vi "BK Precision 9115.vi"() -> ()   [LabVIEW 2020]
uses:
  LabVIEW 2020 Toolkits/toolkits_lv2020_32bit/Synchronization.llb/SynchRefs_SetGet.ctl
  LabVIEW 2020 Toolkits/VI Server Toolkit/VI Server Libraries/VI Server_Set Controls.llb/Set STR Control.vi
  LabVIEW 2020 Toolkits/VI Server Toolkit/VI Server Libraries/VI Server_SetControl.llb/VI Server_BOOL_Set.vi
  LabVIEW 2020 Toolkits/VI Server Toolkit/VI Server Toolkit LV2013.lvlib
panel:
  out "System.Message":string caption="System Message"
  in  "Help":bool
  in  "FP.Hide":bool caption="FrontPanel.Hide"
  in  "EXIT":bool
  in  "error in":errorcluster
  in  "Tab.Main":T1(tab)
  out "Indicator.List.Running":bool
  in  "Indicator.OVP.Level.Measured":dbl caption="Vovp =" format="%0.3f V"
  in  "Indicator.Power.Measured":dbl format="%0.1fW"
  in  "Indicator.Current.Measured":dbl format="%0.3fA"
  in  "Indicator.Voltage.Measured":dbl format="%0.3fV"
  out "Indicator.Prot":bool
  out "Indicator.Trig":bool
  out "Indicator.Error":bool
  out "Indicator.Addr":bool
  out "Indicator.Rmt":bool
  out "Indicator.CC":bool
  out "Indicator.Output.Enabled":bool
  out "Indicator.CV":bool
  in  "OVP.Delay":dbl=0.001 caption="OVP.Delay.DUP" min=0.001 max=0.6 format="%0.3f sec"
  in  "OVP.Level":dbl caption="OVP.Level.DUP" min=0.0 max=80.0 format="%0.3f V"
  in  "Output.Amps":dbl caption="Output.Amps.DUP" min=0.0 max=80.0 format="%0.3f A"
  in  "Output.Volts":dbl caption="Output.Volts.DUP" min=0.0 max=80.0 format="%0.3f V"
  in  "*RST":bool
  in  "LOCAL":bool
  in  "OVP.Clear":bool
  in  "OVP.Enable":bool
  in  "OVP.Delay.DUP":dbl(knob)=0.001 caption="Protection Delay (sec)" min=0.001 max=0.6 scale=0.0..0.6
  in  "OVP.Level.DUP":dbl(knob) caption="Volts" min=0.0 max=80.0 scale=0.0..80.0
  in  "Output.Enable":bool
  in  "Output.Amps.DUP":dbl(knob) caption="Current Limit (Amp)" scale=0.0..60.0
  in  "Output.Volts.DUP":dbl(knob) caption="Volts" min=0.0 max=80.0 scale=0.0..80.0
  in  "Sequence.ActiveSteps":bool[](array[boolean]) caption="Active Steps"
  in  "List.LinkedSequences":bool[](array[boolean]) caption="Linked Sequences"
  in  "List.File.RUN":bool
  in  "Sequence.Load":bool
  in  "Sequence.Save":bool caption="List.File.Save"
  in  "Sequence.RepeatCount":u16[](array[numeric]) caption="Sequence Repeat Count" min=1
  in  "List.RepeatCount":u16=1 caption="List Repeat Count" min=1
  in  "List.PowerLimit":dbl=1.0 caption="List Power Limit" min=1.0 max=1200.0 format="%0.2f W"
  in  "List.File.Load":bool
  in  "List.File.Save":bool
  in  "List.File":u16=1 caption="List File" min=1 max=10
  in  "Sequence.Number":u16=1 caption="Sequence Number" min=1 max=10
  in  "Step.Parameters":T2(array[cluster]) caption="Step Parameters" {"Step.Slope" min=0.01 max=65.535 format="%0.2f sec"; "Step.Width" min=0.001 max=65.535 format="%0.3f sec"; "Step.Current" format="%0.3f A"; "Step.Voltage" format="%0.3f V"}
  out "Sequence.Graph":cluster{i32[], dbl[]}[](graph)
  out "VISA.Messages.Errors":string[](array[string]) caption="VISA Messages Errors"
  in  "Measurements.AutoUpdate.Disable":bool
  in  "Measurements.UpdateRate":u32=100 caption="Measurements Update Rate" min=100 max=100000 format="%.0f msec"
  in  "VISA.Command2.Write":bool
  in  "VISA.Command2":string caption="Command"
  in  "VISA.Command.Write":bool
  in  "VISA.Command":string caption="Command"
  out "VISA.InstrumentResponce":string caption="Instrument Responce"
  in  "VISA.ResourceName":refnum<visa-resource-name>="BK_PRECISION_9115" caption="VISA Rresource Name"
  in  "UDP.Test.String2.Send":bool
  in  "UDP.Test.String2":string caption="UDP: Test String 2"
  in  "UDP.Port.Receiver":u16=58433 caption="UDP: Port.Receiver"
  in  "UDP.Port.Read":u16=58432 caption="UDP: Port.Read"
  in  "UDP.LocalPort.Write":u16=58434 caption="UDP: Local Port.Write"
  in  "UDP.IP.Address":string="234.5.6.7" caption="UDP: IP Address"
  in  "UDP.Test.String1.Send":bool
  in  "UDP.Test.String1":string caption="UDP: Test String 1"
  in  "UDP.Responce.String.Monitor":bool
  out "UDP.Responce.String":string caption="UDP: Responce String"
  in  "VI.WindowsTitle":string caption="Windows Title"
  out "error out":errorcluster={"status"=TRUE, "code"=1055, "source"="Property Node in VI Server Toolkit LV2013.lvlib:VI server_Set Control Value from String Format.vi:5200001->DMM6500_UDP_ExecEng_Instruction_APPLY.vi->DMM6500_UDP_MAIN.vi->Keithley2100.vi"}
  # "OVERVOLTAGE"
  # "OUTPUT"
  # "Seqience Setup"
  # "Step #         Voltage              Current                  Width                     Slope"
  # "1\n\n\n\n2\n\n\n\n3\n\n\n4\n\n\n\n5\n\n\n\n6\n\n\n\n7\n\n\n8\n\n\n\n9\n\n\n\n10"
  # "1       2       3       4       5      6       7      8       9      10"
  # "1       2       3       4       5      6       7      8       9      10"
  # "1"
  # "2"
  # "3"
  # "4"
  # "5"
  # "6"
  # "7"
  # "8"
  # "9"
  # "10"
  # "Multicast IP addresses must be in the 224.0.0.0 to 239.255.255.255 range."
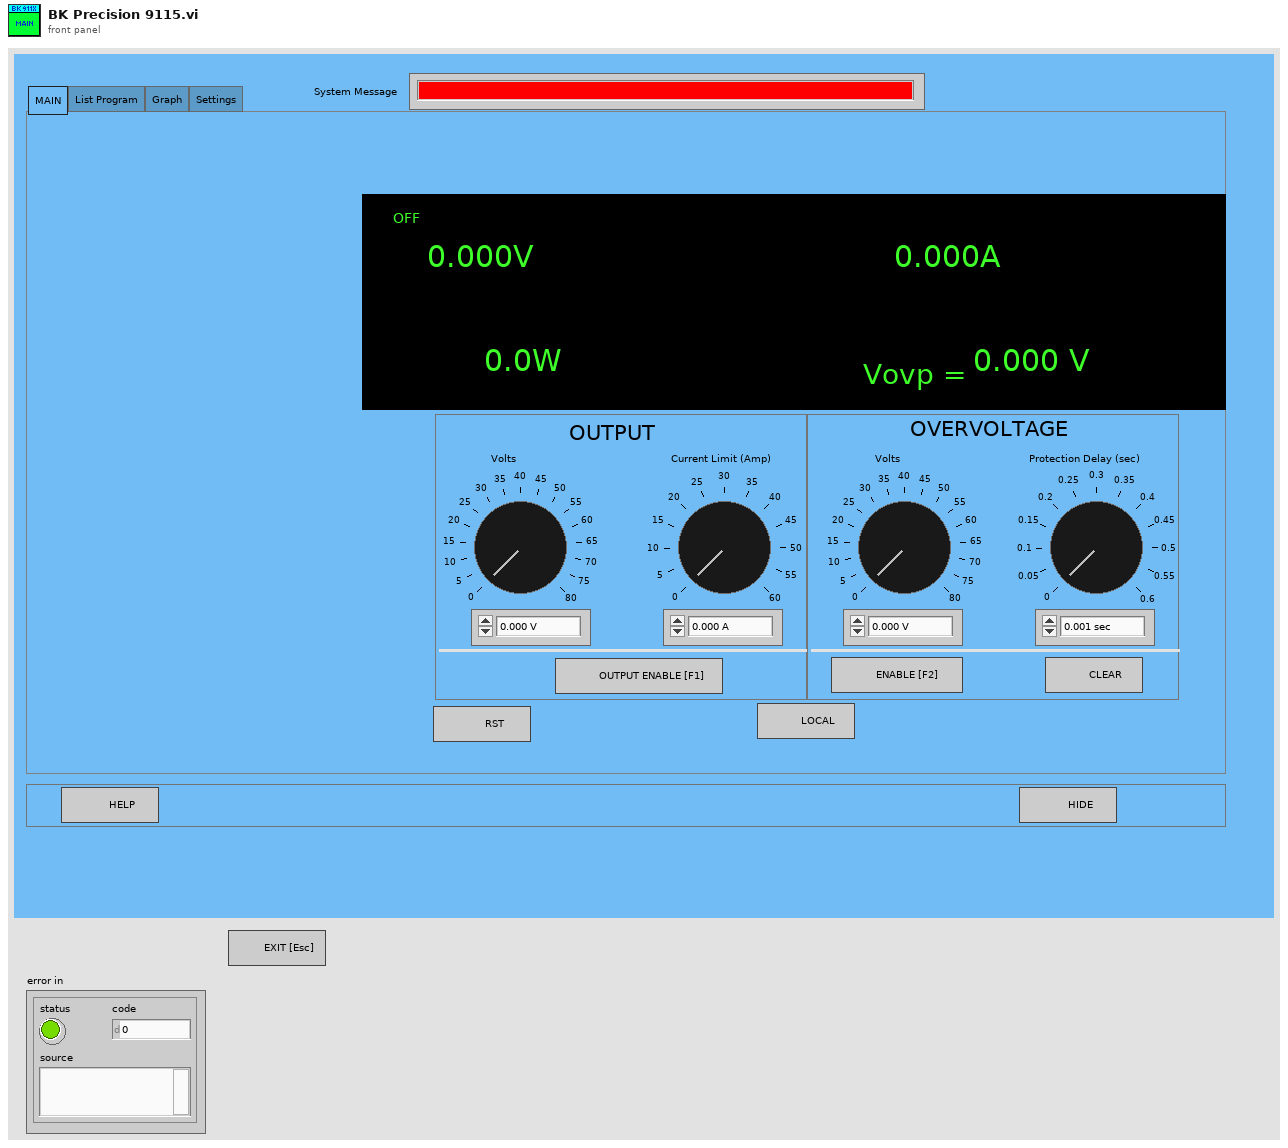
[diagram p1: front panel]
types:
  T1 = enum32{"MAIN", "List Program", "Graph", "Settings"}
  T2 = cluster{"Step.Voltage":dbl, "Step.Current":dbl, "Step.Width":dbl, "Step.Slope":dbl}[]
  T3 = typedef "VI Server_RefsCluster.ctl" = cluster{"Labels":string[], "Refs":refnum<vi>[], "VI Ref":refnum<vi>}
  T4 = typedef "SynchRefs_SetGet.ctl" = enum16{"Set", "Get"}
  T5 = typedef "Semaphore RefNum" = refnum<k1>
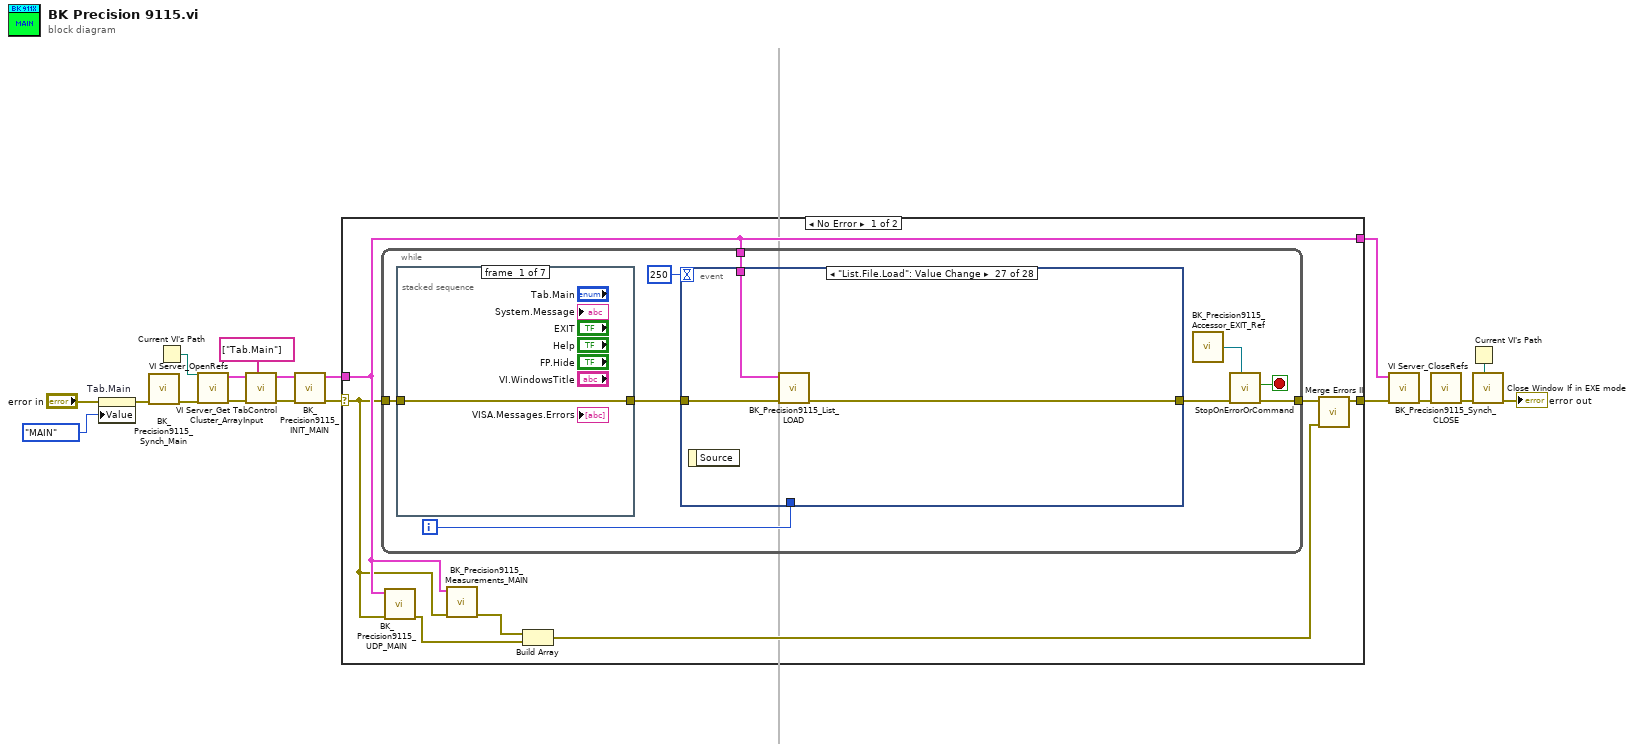
[diagram p0: block diagram]
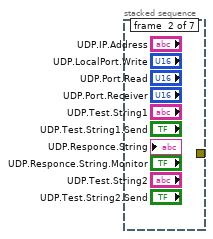
[diagram p2: hidden frame]
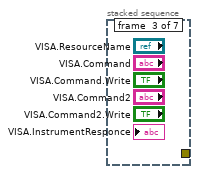
[diagram p3: hidden frame]
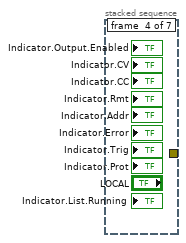
[diagram p4: hidden frame]
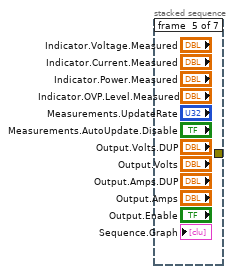
[diagram p5: hidden frame]
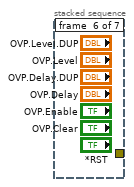
[diagram p6: hidden frame]
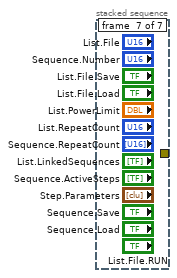
[diagram p7: hidden frame]
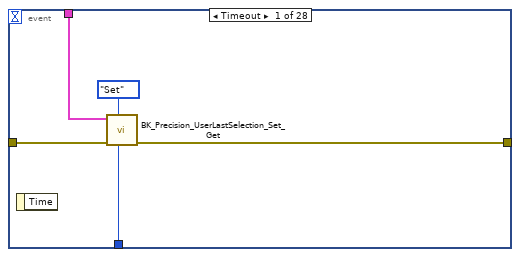
[diagram p8: hidden frame]
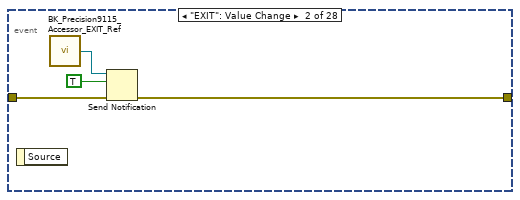
[diagram p9: hidden frame]
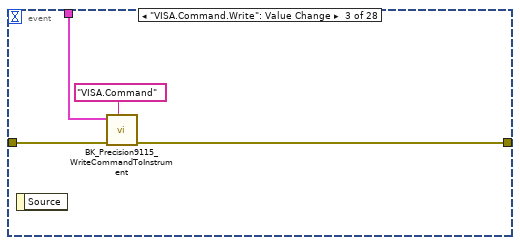
[diagram p10: hidden frame]
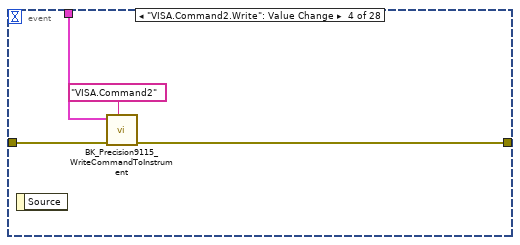
[diagram p11: hidden frame]
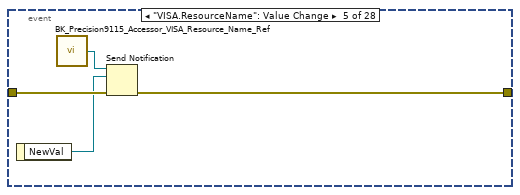
[diagram p12: hidden frame]
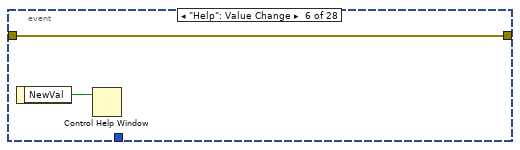
[diagram p13: hidden frame]
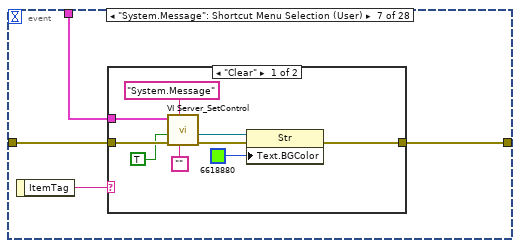
[diagram p14: hidden frame]
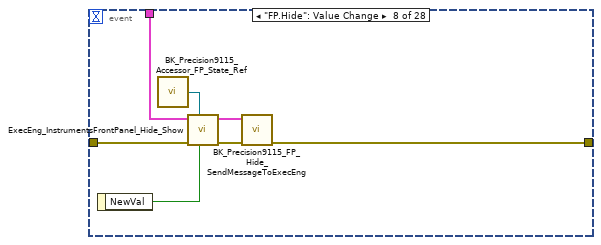
[diagram p16: hidden frame]
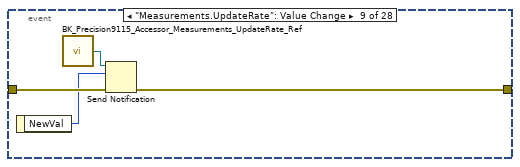
[diagram p17: hidden frame]
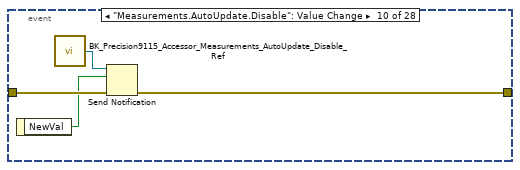
[diagram p18: hidden frame]
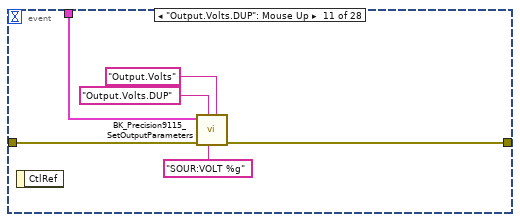
[diagram p19: hidden frame]
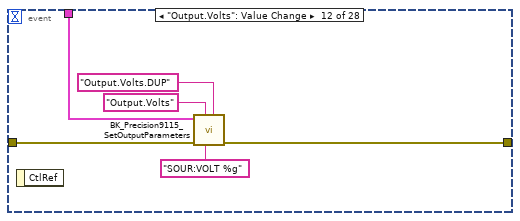
[diagram p20: hidden frame]
diagram:
  n1 = property on="Tab.Main" class="TabCtl (strict)"(error in="error in", "Value"=T1."MAIN" ("Tab.Main")) -> (error out=w2:errorcluster)  [unwired: 1 in, 1 out]
  n2 = call "BK_Precision9115_Synch_Main.vi"("error in"=w2) -> ("error out"=w15:errorcluster)  [unwired: 10 in]
  n3 = Current VI's Path() -> (path=w17:path)
  n4 = call "VI Server_OpenRefs.vi"("error in"=w15, "VI Path"=w17) -> ("error out"=w14:errorcluster, "VI Server.RefsCluster"=w16:T3)  [unwired: 8 in]
  n5 = call "VI Server_Get TabControl Cluster_ArrayInput.vi"("TabControl Labels[]"=string[] ["Tab.Main"], "error in"=w14, "VI Server Cluster"=w16) -> ("error out"=w9:errorcluster, "VI Server Cluster.OUT"=w8:T3)  [unwired: 7 in]
  n6 = call "BK_Precision9115_INIT_MAIN.vi"("error in (no error)"=w9, "VI Server Cluster"=w8) -> ("error out"=w7:errorcluster, "VI Server Cluster DUP"=w5:T3)  [unwired: 8 in]
  n7 = case shown="No Error" w7 {
    selector: w7 -> [w22 w189]
    tunnel: [w24 w189] -> w6
    tunnel: w5 -> [w23 w188]
    tunnel: [w23 w188] -> w4
    frame No Error {
      n8 = while {
        tunnel: w22 -> [w34]
        tunnel: w23 -> [w31]
        tunnel: [w27] -> w25
        i -> [w30]
        stop <- w26 stop-if-true
        n9 = stacked-sequence {
          tunnel: w34 -> [w35 _ _ _ _ _ _]
          tunnel: [w35 _ _ _ _ _ _] -> w32
          frame #0 {
          }
          frame #1 {
          }
          frame #2 {
          }
          frame #3 {
          }
          frame #4 {
          }
          frame #5 {
          }
          frame #6 {
          }
        }
        n10 = event shown="[26] \"List.File.Load\": Value Change" {
          selector: _ -> [_ _ _ _ _ _ _ _ _ _ _ _ _ _ _ _ _ _ _ _ _ _ _ _ _ _ _ _]
          dyn-events: _ -> [_ _ _ _ _ _ _ _ _ _ _ _ _ _ _ _ _ _ _ _ _ _ _ _ _ _ _ _]
          timeout: 250 -> [_ _ _ _ _ _ _ _ _ _ _ _ _ _ _ _ _ _ _ _ _ _ _ _ _ _ _ _]
          tunnel: w32 -> [w40 w44 w48 w52 w56 w57 w61 w79 w83 w87 w92 w98 w104 w110 w114 w120 w126 w132 w138 w143 w146 w159 w171 w174 w177 w180 w183 w187]
          tunnel: w31 -> [w39 _ w47 w51 _ _ w59 w77 _ _ w91 w97 w103 w109 w113 w119 w125 w131 w137 w141 w144 w161 w169 w173 w175 w179 w181 w186]
          tunnel: [w36 w42 w46 w50 w53 w57 w60 w74 w80 w85 w93 w99 w105 w111 w115 w121 w127 w133 w139 w142 w147 w163 w170 w172 w176 w178 w182 w185] -> w28
          tunnel: w30 -> [w38 _ _ _ _ _ _ _ _ _ _ _ _ _ _ _ _ _ _ _ _ _ _ _ _ _ _ _]
          event Timeout {
            n11 = event-data() -> ()  [unwired: 1 in, 1 out]
            n12 = call "BK_Precision_UserLastSelection_Set_Get.vi"("LoopCounter"=w38, "SynchRefs.Set/Get"=SynchRefs_SetGet."Set", "error in"=w40, "VI Server.RefsCluster"=w39) -> ("error out"=w36:errorcluster)  [unwired: 6 in, 1 out]
          }
          event "EXIT": Value Change {
            n13 = event-data() -> ()  [unwired: 1 in, 1 out]
            n14 = call "BK_Precision9115_Accessor_EXIT_Ref.vi"() -> ("EXIT"=w43:refnum<notifier>)  [unwired: 6 in]
            n15 = Send Notification(notification=TRUE, notifier=w43, error in (no error)=w44) -> (error out=w42:errorcluster)  [unwired: 1 out]
          }
          event "VISA.Command.Write": Value Change {
            n16 = event-data() -> ()  [unwired: 1 in, 1 out]
            n17 = call "BK_Precision9115_WriteCommandToInstrument.vi"("Control.Label"="VISA.Command", "error in (no error)"=w48, "VI Server Cluster"=w47) -> ("error out"=w46:errorcluster)  [unwired: 8 in]
          }
          event "VISA.Command2.Write": Value Change {
            n18 = event-data() -> ()  [unwired: 1 in, 1 out]
            n19 = call "BK_Precision9115_WriteCommandToInstrument.vi"("Control.Label"="VISA.Command2", "error in (no error)"=w52, "VI Server Cluster"=w51) -> ("error out"=w50:errorcluster)  [unwired: 8 in]
          }
          event "VISA.ResourceName": Value Change {
            n20 = event-data() -> ("NewVal"=w54:refnum<visa-resource-name>)  [unwired: 1 in]
            n21 = call "BK_Precision9115_Accessor_VISA_Resource_Name_Ref.vi"() -> ("VISA resource name"=w55:refnum<notifier>)  [unwired: 6 in]
            n22 = Send Notification(notification=w54, notifier=w55, error in (no error)=w56) -> (error out=w53:errorcluster)  [unwired: 1 out]
          }
          event "Help": Value Change {
            n23 = event-data() -> ("NewVal"=w58:bool)  [unwired: 1 in]
            n24 = Control Help Window(1:w58) -> ()  [unwired: 1 in]
          }
          event "System.Message": Shortcut Menu Selection (User) {
            n25 = event-data() -> ("ItemTag"=w62:string)  [unwired: 1 in]
            n26 = case shown="\"Clear\"" w62 {
              tunnel: w61 -> [w67 w72]
              tunnel: [w68 w72] -> w60
              tunnel: w59 -> [w65 _]
              frame "Clear" {
                n27 = call-poly "VI Server_SetControl.vi"("New Value"="", "Label"="System.Message", "error in"=w67, "Single Instance (T)"=TRUE ("SingleInstance"), "VI Server Cluster"=w65) -> ("error out"=w70:errorcluster, "Control Ref"=w71:refnum<vi>)  [unwired: 4 in, 1 out]
                n28 = property class="Str"(reference=w71, error in=w70, "Text.BGColor"=u32 6618880) -> (error out=w68:errorcluster)  [unwired: 1 out]
              }
              frame "", Default {
              }
            }
          }
          event "FP.Hide": Value Change {
            n29 = event-data() -> ("NewVal"=w78:bool)  [unwired: 1 in]
            n30 = call "BK_Precision9115_Accessor_FP_State_Ref.vi"() -> ("FP.State"=w76:refnum<notifier>)  [unwired: 6 in]
            n31 = call "ExecEng_InstrumentsFrontPanel_Hide_Show.vi"("FP.Hide/Show"=w78, "FP.State"=w76, "error in (no error)"=w79, "VI Server Cluster"=w77) -> ("error out"=w75:errorcluster, "VI Server Cluster DUP"=w73:T3)  [unwired: 6 in]
            n32 = call "BK_Precision9115_FP_Hide_SendMessageToExecEng.vi"("error in (no error)"=w75, "VI Server Cluster"=w73) -> ("error out"=w74:errorcluster)  [unwired: 9 in]
          }
          event "Measurements.UpdateRate": Value Change {
            n33 = event-data() -> ("NewVal"=w81:u32)  [unwired: 1 in]
            n34 = call "BK_Precision9115_Accessor_Measurements_UpdateRate_Ref.vi"() -> ("Measurements.UpdateRate"=w82:refnum<notifier>)  [unwired: 6 in]
            n35 = Send Notification(notification=w81, notifier=w82, error in (no error)=w83) -> (error out=w80:errorcluster)  [unwired: 1 out]
          }
          event "Measurements.AutoUpdate.Disable": Value Change {
            n36 = event-data() -> ("NewVal"=w86:bool)  [unwired: 1 in]
            n37 = call "BK_Precision9115_Accessor_Measurements_AutoUpdate_Disable_Ref.vi"() -> ("Measurements.AutoUpdate.Disable"=w84:refnum<notifier>)  [unwired: 6 in]
            n38 = Send Notification(notification=w86, notifier=w84, error in (no error)=w87) -> (error out=w85:errorcluster)  [unwired: 1 out]
          }
          event "Output.Volts.DUP": Mouse Up {
            n39 = event-data() -> ()  [unwired: 1 in, 1 out]
            n40 = call "BK_Precision9115_SetOutputParameters.vi"("DuplicateControl.Label"="Output.Volts" ("Control.Label"), "Command.Template"="SOUR:VOLT %g" ("Set Voltage"), "Control.Label"="Output.Volts.DUP", "error in (no error)"=w92, "VI Server Cluster"=w91) -> ("error out"=w93:errorcluster)  [unwired: 5 in, 1 out]
          }
          event "Output.Volts": Value Change {
            n41 = event-data() -> ()  [unwired: 1 in, 1 out]
            n42 = call "BK_Precision9115_SetOutputParameters.vi"("DuplicateControl.Label"="Output.Volts.DUP" ("Control.Label"), "Command.Template"="SOUR:VOLT %g" ("Set Voltage"), "Control.Label"="Output.Volts", "error in (no error)"=w98, "VI Server Cluster"=w97) -> ("error out"=w99:errorcluster)  [unwired: 5 in, 1 out]
          }
          event "Output.Amps.DUP": Mouse Up {
            n43 = event-data() -> ()  [unwired: 1 in, 1 out]
            n44 = call "BK_Precision9115_SetOutputParameters.vi"("DuplicateControl.Label"="Output.Amps" ("Control.Label"), "Command.Template"="SOUR:CURR %g" ("Set Voltage"), "Control.Label"="Output.Amps.DUP", "error in (no error)"=w104, "VI Server Cluster"=w103) -> ("error out"=w105:errorcluster)  [unwired: 5 in, 1 out]
          }
          event "Output.Amps": Value Change {
            n45 = event-data() -> ()  [unwired: 1 in, 3 out]
            n46 = call "BK_Precision9115_SetOutputParameters.vi"("DuplicateControl.Label"="Output.Amps.DUP" ("Control.Label"), "Command.Template"="SOUR:CURR %g" ("Set Voltage"), "Control.Label"="Output.Amps", "error in (no error)"=w110, "VI Server Cluster"=w109) -> ("error out"=w111:errorcluster)  [unwired: 5 in, 1 out]
          }
          event "Output.Enable": Value Change {
            n47 = event-data() -> ("NewVal"=w112:bool)  [unwired: 1 in]
            n48 = call "BK_Precision9115_Output_ENABLE.vi"("Output.Enable"=w112, "error in (no error)"=w114, "VI Server Cluster"=w113) -> ("error out"=w115:errorcluster)  [unwired: 8 in]
          }
          event "OVP.Level.DUP": Mouse Up {
            n49 = event-data() -> ()  [unwired: 1 in, 1 out]
            n50 = call "BK_Precision9115_SetOutputParameters.vi"("DuplicateControl.Label"="OVP.Level" ("Control.Label"), "Command.Template"="SOUR:VOLT:PROT %g" ("Set Voltage"), "Control.Label"="OVP.Level.DUP", "error in (no error)"=w120, "VI Server Cluster"=w119) -> ("error out"=w121:errorcluster)  [unwired: 5 in, 1 out]
          }
          event "OVP.Level": Value Change {
            n51 = event-data() -> ()  [unwired: 1 in, 1 out]
            n52 = call "BK_Precision9115_SetOutputParameters.vi"("DuplicateControl.Label"="OVP.Level.DUP" ("Control.Label"), "Command.Template"="SOUR:VOLT:PROT %g" ("Set Voltage"), "Control.Label"="OVP.Level", "error in (no error)"=w126, "VI Server Cluster"=w125) -> ("error out"=w127:errorcluster)  [unwired: 5 in, 1 out]
          }
          event "OVP.Delay.DUP": Mouse Up {
            n53 = event-data() -> ()  [unwired: 1 in, 1 out]
            n54 = call "BK_Precision9115_SetOutputParameters.vi"("DuplicateControl.Label"="OVP.Delay" ("Control.Label"), "Command.Template"="SOUR:VOLT:PROT:DEL %g" ("Set Voltage"), "Control.Label"="OVP.Delay.DUP", "error in (no error)"=w132, "VI Server Cluster"=w131) -> ("error out"=w133:errorcluster)  [unwired: 5 in, 1 out]
          }
          event "OVP.Delay": Value Change {
            n55 = event-data() -> ()  [unwired: 1 in, 1 out]
            n56 = call "BK_Precision9115_SetOutputParameters.vi"("DuplicateControl.Label"="OVP.Delay.DUP" ("Control.Label"), "Command.Template"="SOUR:VOLT:PROT:DEL %g" ("Set Voltage"), "Control.Label"="OVP.Delay", "error in (no error)"=w138, "VI Server Cluster"=w137) -> ("error out"=w139:errorcluster)  [unwired: 5 in, 1 out]
          }
          event "OVP.Enable": Value Change {
            n57 = event-data() -> ("NewVal"=w140:bool)  [unwired: 1 in]
            n58 = call "BK_Precision9115_OverVoltageProtection_Enable.vi"("OVP.Enable"=w140, "error in (no error)"=w143, "VI Server Cluster"=w141) -> ("error out"=w142:errorcluster)  [unwired: 8 in]
          }
          event "LOCAL": Value Change {
            n59 = event-data() -> ("NewVal"=w145:bool)  [unwired: 1 in]
            n60 = call "BK_Precision9115_Control_Local.vi"("Local"=w145, "error in (no error)"=w146, "VI Server Cluster"=w144) -> ("error out"=w147:errorcluster)  [unwired: 8 in]
          }
          event "*RST": Value Change {
            w152 = "*RST;*CLS" ("Set Voltage")
            n61 = event-data() -> ()  [unwired: 1 in, 1 out]
            n62 = call-poly "VI Server_SetControl.vi"("Data"=FALSE, "Control.Label"="*RST" ("Set Voltage"), "error in"=w159, "SingleInstance"=TRUE, "VI Server.RefsCluster"=w161) -> ("error out"=w160:errorcluster, "VI Server.RefsCluster.DUP"=w154:T3)  [unwired: 4 in, 1 out]
            n63 = call "BK_Precision9115_Accessor_VISA_Resource_Name_Ref.vi"() -> ("VISA resource name"=w168:refnum<notifier>)  [unwired: 6 in]
            n64 = call "BK_Precision9115_Accessor_Command.Sem_Ref.vi"() -> ("Command.Sem"=w164:T5)  [unwired: 6 in]
            n65 = call "Semaphore_Acquire.vi"("error in"=w160, "SemaphoreRef"=w164) -> ("error out"=w166:errorcluster)  [unwired: 8 in, 1 out]
            n66 = Get Notifier Status(notifier=w168, error in (no error)=w166) -> (current notification=w167:refnum<visa-resource-name>, error out=w165:errorcluster)  [unwired: 3 out]
            n67 = call "VISA WriteMod.vi"("error in"=w165, "String"=w152, "VISA resource name"=w167) -> ("error out"=w155:errorcluster, "VISA resource name DUP"=w153:refnum<visa-resource-name>)  [unwired: 6 in, 1 out]
            n68 = Current VI's Path() -> (path=w151:path)
            n69 = call "BK_Precision9115_ErrorHandler.vi"("Calling VI.Path"=w151, "Command"=w152, "VISA Refnum"=w153, "error in (no error)"=w155, "VI Server.RefsCluster"=w154) -> ("error out"=w149:errorcluster)  [unwired: 4 in, 2 out]
            n70 = call "BK_Precision9115_Accessor_Command.Sem_Ref.vi"() -> ("Command.Sem"=w162:T5)  [unwired: 6 in]
            n71 = call "Error 1073807246_SerialInterface_VISA resourceIsValidButNotAccessable.vi"("ShowError"=TRUE, "error in"=w149) -> ("error out"=w148:errorcluster)  [unwired: 12 in, 1 out]
            n72 = call "Semaphore_Release.vi"("error in"=w148, "SemaphoreRef"=w162) -> ("error out"=w163:errorcluster)  [unwired: 8 in, 1 out]
          }
          event "OVP.Clear": Value Change {
            n73 = event-data() -> ()  [unwired: 1 in, 1 out]
            n74 = call "BK_Precision9115_OVP_CLEAR.vi"("error in (no error)"=w171, "VI Server Cluster"=w169) -> ("error out"=w170:errorcluster)  [unwired: 8 in, 1 out]
          }
          event "Sequence.Save": Value Change {
            n75 = event-data() -> ()  [unwired: 1 in, 1 out]
            n76 = call "BK_Precision9115_Sequence_SAVE.vi"("error in (no error)"=w174, "VI Server Cluster"=w173) -> ("error out"=w172:errorcluster)  [unwired: 9 in]
          }
          event "Sequence.Load": Value Change {
            n77 = event-data() -> ()  [unwired: 1 in, 1 out]
            n78 = call "BK_Precision9115_Sequence_LOAD.vi"("error in (no error)"=w177, "VI Server Cluster"=w175) -> ("error out"=w176:errorcluster)  [unwired: 9 in]
          }
          event "List.File.Save": Value Change {
            n79 = event-data() -> ()  [unwired: 1 in, 1 out]
            n80 = call "BK_Precision9115_List_SAVE.vi"("error in (no error)"=w180, "VI Server Cluster"=w179) -> ("error out"=w178:errorcluster)  [unwired: 9 in]
          }
          event "List.File.Load": Value Change {
            n81 = event-data() -> ()  [unwired: 1 in, 1 out]
            n82 = call "BK_Precision9115_List_LOAD.vi"("error in (no error)"=w183, "VI Server Cluster"=w181) -> ("error out"=w182:errorcluster)  [unwired: 9 in]
          }
          event "List.File.RUN": Value Change {
            n83 = event-data() -> ("NewVal"=w184:bool)  [unwired: 1 in]
            n84 = call "BK_Precision9115_List_RUN.vi"("List.File.RUN"=w184, "error in (no error)"=w187, "VI Server Cluster"=w186) -> ("error out"=w185:errorcluster)  [unwired: 8 in]
          }
        }
        n85 = call "BK_Precision9115_Accessor_EXIT_Ref.vi"() -> ("EXIT"=w29:refnum<notifier>)  [unwired: 6 in]
        n86 = call "StopOnErrorOrCommand.vi"("STOP"=w29, "error in (no error)"=w28) -> ("error out"=w27:errorcluster, "STOP"=w26:bool)  [unwired: 8 in]
      }
      n87 = call "BK_Precision9115_UDP_MAIN.vi"("error in (no error)"=w22, "VI Server.RefsCluster"=w23) -> ("error out"=w20:errorcluster)  [unwired: 9 in]
      n88 = call "BK_Precision9115_Measurements_MAIN.vi"("error in (no error)"=w22, "VI Server.RefsCluster"=w23) -> ("error out"=w21:errorcluster)  [unwired: 9 in]
      n89 = Build Array(w21, w20) -> (w19:errorcluster[])
      n90 = call "Merge Errors II.vi"("error array in"=w19, "error in 1 (no error)"=w25) -> ("error out.DUP"=w24:errorcluster)  [unwired: 4 in, 1 out]
    }
    frame Error {
    }
  }
  n91 = call "VI Server_CloseRefs.vi"("error in"=w6, "VI Server.RefsCluster"=w4) -> ("error out"=w12:errorcluster)  [unwired: 9 in]
  n92 = call "BK_Precision9115_Synch_CLOSE.vi"("error in"=w12) -> ("error out"=w11:errorcluster)  [unwired: 10 in]
  n93 = Current VI's Path() -> (path=w18:path)
  n94 = call "Close Window If in EXE mode.vi"("TopLevelVI Path"=w18, "error in"=w11) -> ("error out"=→"error out":errorcluster)  [unwired: 9 in]
